vi "Initialize Truck.vi"(6 "Interior cargo capacity":dbl=67.0, 8 "model":string="pickup", 9 "make":string="Company B", 10 "Bed cargo capacity":dbl=64.4, 11 "truck in":refnum<class "Truck.lvclass">) -> (3 "truck out":refnum<class "Truck.lvclass">)   [LabVIEW 2023, in "Truck.lvclass"]
doc: "This method initializes the data members of the class \"Truck.\""
uses:
  Truck.lvclass
  c:/dev/_r/4/eng/lv-core/lvpostprocessingd/lv_mc_x86_64/dist_i386/examples/Object-Oriented Programming/Custom Probes/Vehicle/Vehicle.lvclass
  Truck.lvclass/Truck.ctl
  Vehicle/Vehicle.lvclass
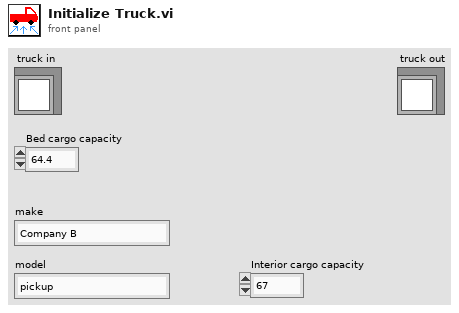
[diagram p1: front panel]
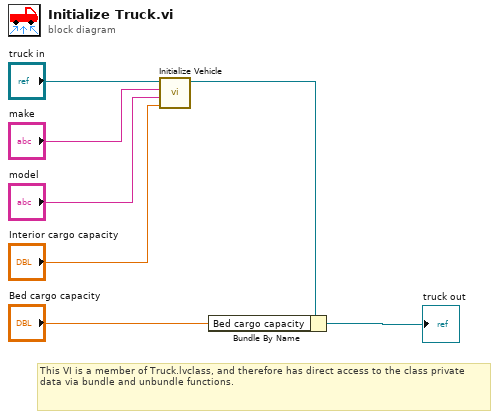
[diagram p0: block diagram]
diagram:
  # "This VI is a member of Truck.lvclass, and therefore has direct access to the class private data via bundle and unbundle functions."
  n1 = call "Initialize Vehicle.vi"("Interior cargo capacity"="Interior cargo capacity", "model"="model", "make"="make", "vehicle in"="truck in") -> ("vehicle out"=w4:refnum<class "Truck.lvclass">)  [unwired: 7 in]
  n2 = Bundle By Name(cluster=w4, "Bed cargo capacity"="Bed cargo capacity") -> (→"truck out":refnum<class "Truck.lvclass">)
